vi "Updater Convert TDMS File 5.0 to 5.1 Prompted Input.vi"(6 "Connection Refnum In":T1, 7 "TDMS Path In":path, 8 "error in (no error)":errorcluster, 11 "TDMS File Ref":refnum<k34>) -> (0 "error out":errorcluster, 3 "TDMS File Ref":refnum<k34>, 4 "Connection Refnum Out":T1, 5 "TDMS Path Out":path)   [LabVIEW 2011]
uses:
  Summitek EXT/ODBC/SQL Controls/Connection Refnum.ctl
  server/database/Fields/Field Record.ctl
  server/database/Fields/Field DataTypes.ctl
  server/database/Fields/Field NextItem.ctl
  server/database/Fields/Field Order By.ctl
  Summitek EXT/OpenG EXT/file/file.llb/Convert File Extension (Path)__ogtk.vi
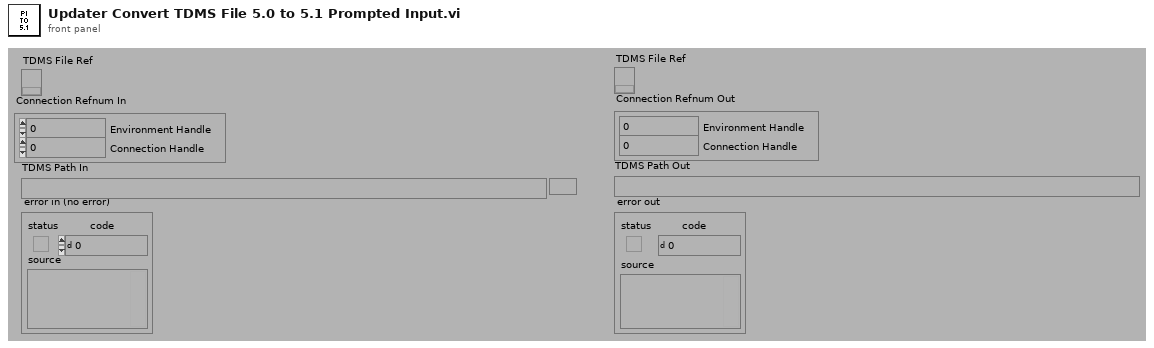
[diagram p1: front panel]
types:
  T1 = typedef "Connection Refnum.ctl" = cluster{"Environment Handle":i32, "Connection Handle":i32}
  T2 = enum16{"open", "open or create", "create or replace", "create", "open (read-only)"}
  T3 = typedef "Field Record.ctl" = cluster{"ixField":i32, "iSequenceOrder":i32, "sxFieldId":string, "sxSequenceId":string, "sDisplayName":string, "sValue":string, "sUnits":string, "nDataType":T4, "nNextItem":T5, "fSystem":bool, "fSystemValue":bool, "fRequired":bool, "fSetAtTest":bool, "fTestField":bool, "fDeleted":bool, "fIndexed":bool, "fFreeList":bool}
  T4 = typedef "Field DataTypes.ctl" = enum32{"text", "numeric", "list", "timestamp", "boolean"}
  T5 = typedef "Field NextItem.ctl" = enum32{"Reset", "Retain", "Auto-Increment"}
  T6 = typedef "Field Order By.ctl" = enum32{"sxSequenceId", "sxFieldId", "sDisplayName", "sValue", "fSetAtTest", "fRequired", "nNextItem"}
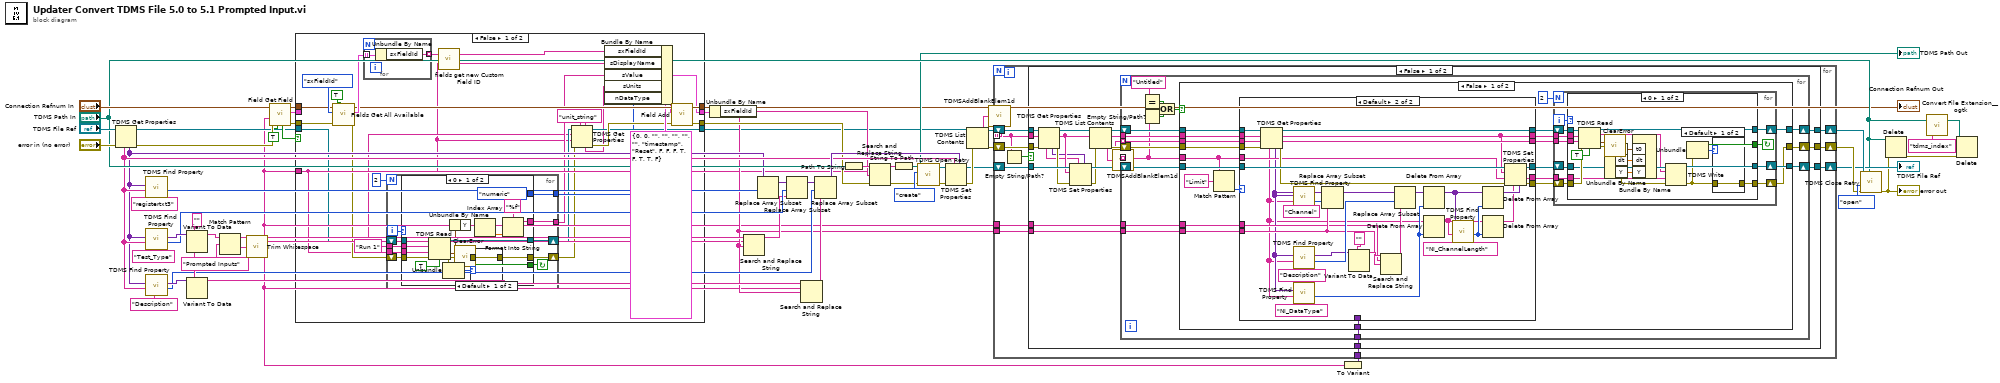
[diagram p0: block diagram]
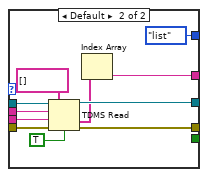
[diagram p3: hidden frame]
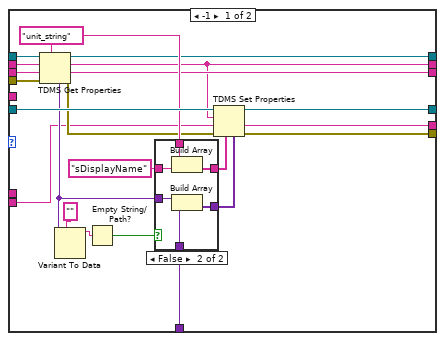
[diagram p5: hidden frame]
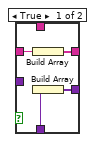
[diagram p6: hidden frame]
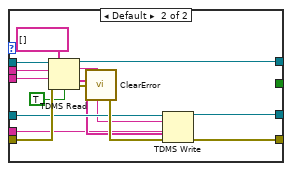
[diagram p8: hidden frame]
diagram:
  w2 = TRUE ("by sDisplayName? (f, by sFieldId)")
  w29 = "" ("element")
  n1 = TDMS Get Properties(8:"error in (no error)", 11:"TDMS File Ref") -> (0:w38:errorcluster, 3:w5:refnum<k34>, 4:w21:variant[], 6:w22:string[])  [unwired: 1 in, 5 out]
  n2 = call "TDMS Find Property.vi"("Property Name"="registertxt3" ("element"), "Property Names"=w22, "Property Values"=w21) -> ("Index"=w19:i32)  [unwired: 5 out]
  n3 = call "TDMS Find Property.vi"("Property Name"="Test_Type" ("element"), "Property Names"=w22, "Property Values"=w21) -> ("Index"=w18:i32, "Property Value"=w40:variant)  [unwired: 4 out]
  n4 = call "TDMS Find Property.vi"("Property Name"="Description" ("element"), "Property Names"=w22, "Property Values"=w21) -> ("Index"=w25:i32, "Property Value"=w30:variant)  [unwired: 4 out]
  n5 = Variant To Data(type=w29, Variant=w40) -> (data=w14:string)  [unwired: 1 in, 1 out]
  n6 = Variant To Data(type=w29, Variant=w30) -> (data=w28:string)  [unwired: 1 in, 1 out]
  n7 = Match Pattern(string=w14, regular expression="Prompted Inputs" ("element")) -> (after substring=w39:string)  [unwired: 4 out]
  n8 = call <vilib>:"Trim Whitespace.vi"("string"=w39) -> ("trimmed string"=w3:string)  [unwired: 1 in]
  n9 = call "Field Get Field.vi"("by sDisplayName? (f, by sFieldId)"=w2, "Include deleted? (F)"=w2, "error in (no error)"=w38, "sFieldId or sDisplayName (\"\")"=w3, "Connection Refnum"="Connection Refnum In") -> ("error out"=w11:errorcluster, "Field"=w36:T3, "Connection Refnum"=w10:T1, "Data Present?"=w12:bool)  [unwired: 1 in, 2 out]
  n10 = case shown="False" w12 {
    tunnel: w36 -> [_ w126]
    tunnel: [w60 w126] -> w6
    tunnel: w11 -> [w81 w127]
    tunnel: w10 -> [w82 w128]
    tunnel: [w75 w128] -> w8
    tunnel: [w74 w127] -> w9
    tunnel: w3 -> [w61 _]
    tunnel: w5 -> [w66 w125]
    tunnel: [w72 w125] -> w4
    frame False {
      w71 = "unit_string" ("string")
      w62 = "Run 1" ("group name in")
      w84 = TRUE
      n11 = call "Fields Get All Available.vi"("Combine All? (f)"=w84, "Include Deleted? (F)"=w84, "error in (no error)"=w81, "Sort by (sxSequenceId)"=Field_Order_By."sxFieldId" ("Sort by (Sequence_ID)"), "Connection Refnum"=w82) -> ("error out"=w63:errorcluster, "System or ALL Combined Fields"=w80:T3[], "Connection Refnum"=w78:T1)  [unwired: 1 in, 3 out]
      n12 = for {
        tunnel: w80 -> [w124] mode=indexing
        tunnel: [w123] -> w79 mode=indexing
        n13 = Unbundle By Name(w124) -> ("sxFieldId"=w123:string)
      }
      n14 = for {
        N: 2 -> [_]
        tunnel: w61 -> [w93]
        tunnel: w62 -> [w92]
        shift-right: [w94] -> w65
        shift-left: w66 -> [w91]
        tunnel: [w88] -> w68
        shift-right: [w86] -> w64
        shift-left: w63 -> [w87]
        tunnel: [w85] -> w67
        i -> [w90]
        stop <- w89 continue-if-true
        n15 = case shown="0" w90 {
          tunnel: [w111 w122] -> w94
          tunnel: w93 -> [w110 w121]
          tunnel: w92 -> [w109 w120]
          tunnel: w91 -> [w108 w119]
          tunnel: [w106 _] -> w89
          tunnel: [Field_DataTypes."numeric" ("nDataType") Field_DataTypes."list" ("nDataType")] -> w88
          tunnel: w87 -> [w104 w115]
          tunnel: [w103 w115] -> w86
          tunnel: [w98 w114] -> w85
          frame 0 {
            n16 = TDMS Read(0:w108, 5:w109, 7:w110, 11:w104, 13:TRUE ("return channels in file order? (F)")) -> (4:w111:refnum<k34>, 10:w97:waveform(dbl), 15:w96:errorcluster)  [unwired: 3 in, 3 out]
            n17 = Unbundle By Name(w97) -> ("Y"=w101:dbl[])
            n18 = call <vilib>:"ClearError.vi"("error in (no error)"=w96) -> ("error out"=w105:errorcluster)
            n19 = Unbundle(w105) -> ("status"=w106:bool, "code"=w107:i32)  [unwired: 1 out]
            n20 = case shown="Default" w107 {
              tunnel: [w112 _] -> w103
              tunnel: w105 -> [w112 _]
              frame Default {
              }
              frame -2525 {
              }
            }
            n21 = Index Array(array=w101) -> (element=w100:dbl)  [unwired: 1 in]
            n22 = Format Into String(format string="%f", w100) -> (resulting string=w98:string)  [unwired: 2 in, 1 out]
          }
          frame Default {
            n23 = TDMS Read(0:w119, 5:w120, 7:w121, 12:string[] [], 13:TRUE ("return channels in file order? (F)")) -> (4:w122:refnum<k34>, 10:w116:string[])  [unwired: 3 in, 4 out]
            n24 = Index Array(array=w116) -> (element=w114:string)  [unwired: 1 in]
          }
        }
      }
      n25 = call "fields get new Custom Field ID.vi"("Existing Field IDs (empty)"=w79) -> ("Custom Field ID"=w76:string)  [unwired: 1 in, 1 out]
      n26 = TDMS Get Properties(5:w71, 7:w71, 8:w64, 9:w61, 10:w62, 11:w65) -> (0:w73:errorcluster, 3:w72:refnum<k34>, 4:w70:string)  [unwired: 3 out]
      n27 = Bundle By Name(cluster=T3 {"ixField"=0, "iSequenceOrder"=0, "sxFieldId"="", "sxSequenceId"="", "sDisplayName"="", "sValue"="", "sUnits"="", "nDataType"=enum."timestamp", "nNextItem"=enum."Reset", "fSystem"=FALSE, "fSystemValue"=FALSE, "fRequired"=FALSE, "fSetAtTest"=TRUE, "fTestField"=FALSE, "fDeleted"=TRUE, "fIndexed"=TRUE, "fFreeList"=FALSE} ("Field Record"), "sxFieldId"=w76, "sDisplayName"=w61, "sValue"=w67, "sUnits"=w70, "nDataType"=w68) -> (w60:T3)
      n28 = call "Field Add.vi"("error in (no error)"=w73, "Field Record"=w60, "Connection Refnum"=w78) -> ("error out"=w74:errorcluster, "Connection Refnum"=w75:T1)  [unwired: 1 in, 6 out]
    }
    frame True {
    }
  }
  "Connection Refnum Out" <- w8
  n29 = Unbundle By Name(w6) -> ("sxFieldId"=w7:string)
  n30 = Search and Replace String(input string=w14, search string=w3, replace string=w7) -> (result string=w13:string)  [unwired: 1 in, 7 out]
  n31 = Replace Array Subset(array=w21, new element=w13, index=w19) -> (w20:variant[])
  n32 = Replace Array Subset(array=w20, new element=w13, index=w18) -> (w27:variant[])
  n33 = Search and Replace String(input string=w28, search string=w3, replace string=w7) -> (result string=w26:string)  [unwired: 1 in, 7 out]
  n34 = Replace Array Subset(array=w27, new element=w26, index=w25) -> (w24:variant[])
  n35 = Path To String(path="TDMS Path In") -> (string=w35:string)
  n36 = Search and Replace String(input string=w35, search string=w3, replace string=w7, error in=w9) -> (result string=w34:string, error out=w33:errorcluster)  [unwired: 6 out]
  n37 = String To Path(string=w34) -> (path=w15:path)
  "TDMS Path Out" <- w15
  n38 = call "TDMS Open Retry.vi"("error in (no error)"=w33, "Operation (0:open)"=T2."create" ("operation (0:open)"), "Path"=w15) -> ("error out"=w53:errorcluster, "TDMS File Ref"=w52:refnum<k34>)  [unwired: 1 in, 6 out]
  n39 = TDMS Set Properties(5:w24, 7:w22, 8:w53, 11:w52) -> (0:w57:errorcluster, 3:w51:refnum<k34>)  [unwired: 4 out]
  n40 = TDMS List Contents(4:w57, 7:w4) -> (0:w56:errorcluster, 2:w1:string[], 3:w50:refnum<k34>)  [unwired: 2 out]
  n41 = call <vilib>:"TDMSAddBlankElem1d.vi"("input string array"=w1) -> ("output string array with blank element at the beginning"=w59:string[])
  n42 = To Variant(anything=w3) -> (Variant=w16:variant)
  n43 = for {
    shift-right: [w137] -> w55
    shift-left: w56 -> [w138]
    tunnel: w59 -> [w136] mode=indexing
    shift-right: [w133] -> w49
    shift-left: w50 -> [w139]
    shift-right: [w132] -> w45
    shift-left: w51 -> [w135]
    tunnel: w16 -> [w131]
    tunnel: w7 -> [w130]
    tunnel: w3 -> [w129]
    n44 = Empty String/Path?(string/path=w136) -> (empty?=w134:bool)
    n45 = case shown="False" w134 {
      tunnel: w139 -> [w161 w318]
      tunnel: w138 -> [w160 w319]
      tunnel: [w153 w319] -> w137
      tunnel: w136 -> [w159 _]
      tunnel: w135 -> [w150 w317]
      tunnel: [w156 w318] -> w133
      tunnel: [w155 w317] -> w132
      tunnel: w131 -> [w143 _]
      tunnel: w130 -> [w142 _]
      tunnel: w129 -> [w141 _]
      frame False {
        n46 = TDMS Get Properties(8:w160, 10:w159, 11:w161) -> (0:w147:errorcluster, 2:w148:string, 3:w158:refnum<k34>, 4:w146:variant[], 6:w145:string[])  [unwired: 1 in, 3 out]
        n47 = TDMS Set Properties(5:w146, 7:w145, 8:w147, 10:w148, 11:w150) -> (0:w149:errorcluster, 3:w151:refnum<k34>)  [unwired: 3 out]
        n48 = TDMS List Contents(4:w149, 6:w148, 7:w158) -> (0:w154:errorcluster, 1:w140:string[], 2:w152:string, 3:w157:refnum<k34>)
        n49 = call <vilib>:"TDMSAddBlankElem1d.vi"("input string array"=w140) -> ("output string array with blank element at the beginning"=w144:string[])
        n50 = for {
          shift-right: [w170] -> w156
          shift-left: w157 -> [w175]
          shift-right: [w172] -> w155
          shift-left: w151 -> [w177]
          shift-right: [w171] -> w153
          shift-left: w154 -> [w176]
          tunnel: w152 -> [w174]
          tunnel: w144 -> [w173] mode=indexing
          tunnel: w144 -> [w164] mode=indexing
          tunnel: w143 -> [w165]
          tunnel: w142 -> [w163]
          tunnel: w141 -> [w162]
          n51 = Equal?(x="Untitled" ("string"), y=w164) -> (x = y?=w167:bool)
          n52 = Empty String/Path?(string/path=w164) -> (empty?=w168:bool)
          n53 = Or(x=w167, y=w168) -> (x .or. y?=w166:bool)
          n54 = case shown="False" w166 {
            tunnel: w177 -> [w198 w315]
            tunnel: w176 -> [w197 w314]
            tunnel: w175 -> [w196 w316]
            tunnel: w174 -> [w195 _]
            tunnel: w173 -> [w194 _]
            tunnel: [w191 w315] -> w172
            tunnel: [w190 w314] -> w171
            tunnel: [w189 w316] -> w170
            tunnel: w164 -> [w183 _]
            tunnel: w165 -> [w188 _]
            tunnel: w163 -> [w180 _]
            tunnel: w162 -> [w179 _]
            frame False {
              n55 = Match Pattern(string=w183, regular expression="Limit") -> (offset past match=w181:i32)  [unwired: 4 out]
              n56 = case shown="Default" w181 {
                tunnel: w198 -> [w220 w265]
                tunnel: w197 -> [w219 w264]
                tunnel: w196 -> [w218 w263]
                tunnel: w195 -> [w217 w262]
                tunnel: w194 -> [w216 w261]
                tunnel: [w215 w260] -> w193
                tunnel: [w214 w259] -> w192
                tunnel: w188 -> [w210 _]
                tunnel: [w203 w257] -> w187
                tunnel: [w202 w256] -> w186
                tunnel: [w201 w255] -> w185
                tunnel: w183 -> [_ w254]
                tunnel: w180 -> [w200 w245]
                tunnel: w179 -> [_ w244]
                tunnel: [w199 w231] -> w178
                frame -1 {
                  w208 = "unit_string" ("string")
                  n57 = TDMS Get Properties(7:w208, 8:w219, 9:w216, 10:w217, 11:w218) -> (0:w204:errorcluster, 1:w203:string, 2:w202:string, 3:w201:refnum<k34>, 4:w207:variant)  [unwired: 2 out]
                  n58 = Variant To Data(type="" ("element"), Variant=w207) -> (data=w212:string)  [unwired: 1 in, 1 out]
                  n59 = Empty String/Path?(string/path=w212) -> (empty?=w211:bool)
                  n60 = case shown="False" w211 {
                    tunnel: [w224 w228] -> w206
                    tunnel: w210 -> [w223 w230]
                    tunnel: [w222 w227] -> w205
                    tunnel: "sDisplayName" ("element") -> [w221 w229]
                    tunnel: w208 -> [_ w226]
                    tunnel: w207 -> [_ w225]
                    frame True {
                      n61 = Build Array(w221) -> (w224:string[])
                      n62 = Build Array(w223) -> (w222:variant[])
                    }
                    frame False {
                      n63 = Build Array(w226, w229) -> (w228:string[])
                      n64 = Build Array(w225, w230) -> (w227:variant[])
                    }
                  }
                  n65 = TDMS Set Properties(5:w205, 7:w206, 8:w204, 9:w200, 10:w202, 11:w220) -> (0:w215:errorcluster, 1:w199:string, 3:w214:refnum<k34>)  [unwired: 1 out]
                }
                frame Default {
                  n66 = TDMS Get Properties(8:w264, 9:w261, 10:w262, 11:w263) -> (0:w258:errorcluster, 1:w257:string, 2:w256:string, 3:w255:refnum<k34>, 4:w239:variant[], 6:w236:string[])  [unwired: 2 out]
                  n67 = call "TDMS Find Property.vi"("Property Name"="Channel" ("element"), "Property Names"=w236, "Property Values"=w239) -> ("Index"=w252:i32)  [unwired: 5 out]
                  n68 = call "TDMS Find Property.vi"("Property Name"="Description" ("element"), "Property Names"=w236, "Property Values"=w239) -> ("Index"=w249:i32, "Property Value"=w247:variant)  [unwired: 4 out]
                  n69 = call "TDMS Find Property.vi"("Property Name"="NI_DataType" ("element"), "Property Names"=w236, "Property Values"=w239) -> ("Index"=w238:i32)  [unwired: 5 out]
                  n70 = Replace Array Subset(array=w239, new element=w245, index=w252) -> (w250:variant[])
                  n71 = Variant To Data(type="" ("element"), Variant=w247) -> (data=w246:string)  [unwired: 1 in, 1 out]
                  n72 = Search and Replace String(input string=w246, search string=w244, replace string=w245) -> (result string=w243:string)  [unwired: 1 in, 7 out]
                  n73 = Replace Array Subset(array=w250, new element=w243, index=w249) -> (w242:variant[])
                  n74 = Delete From Array(array=w242, index=w238) -> (array with subset deleted=w233:variant[])  [unwired: 1 in, 1 out]
                  n75 = Delete From Array(array=w236, index=w238) -> (array with subset deleted=w232:string[])  [unwired: 1 in, 1 out]
                  n76 = call "TDMS Find Property.vi"("Property Name"="NI_ChannelLength" ("element"), "Property Names"=w232, "Property Values"=w233) -> ("Index"=w234:i32)  [unwired: 5 out]
                  n77 = Delete From Array(array=w233, index=w234) -> (array with subset deleted=w237:variant[])  [unwired: 1 in, 1 out]
                  n78 = Delete From Array(array=w232, index=w234) -> (array with subset deleted=w235:string[])  [unwired: 1 in, 1 out]
                  n79 = TDMS Set Properties(5:w237, 7:w235, 8:w258, 9:w254, 10:w256, 11:w265) -> (0:w260:errorcluster, 1:w231:string, 3:w259:refnum<k34>)  [unwired: 1 out]
                }
              }
              n80 = for {
                N: 2 -> [_]
                tunnel: w187 -> [w272]
                tunnel: w186 -> [w271]
                shift-right: [w268] -> w190
                shift-left: w193 -> [w276]
                shift-right: [w274] -> w191
                shift-left: w192 -> [w275]
                shift-right: [w273] -> w189
                shift-left: w185 -> [w270]
                tunnel: w178 -> [w266]
                i -> [w269]
                stop <- w267 continue-if-true
                n81 = case shown="0" w269 {
                  tunnel: w276 -> [w297 w313]
                  tunnel: w275 -> [w295 w311]
                  tunnel: [w293 w308] -> w274
                  tunnel: [w288 w307] -> w268
                  tunnel: [w292 w306] -> w273
                  tunnel: w272 -> [w291 w305]
                  tunnel: w271 -> [w290 w304]
                  tunnel: w270 -> [w289 w303]
                  tunnel: [w285 _] -> w267
                  tunnel: w266 -> [w284 w301]
                  frame 0 {
                    n82 = TDMS Read(0:w289, 5:w290, 7:w291, 11:w297, 13:TRUE ("return channels in file order? (F)")) -> (4:w292:refnum<k34>, 6:w294:string, 10:w283:waveform(dbl), 15:w278:errorcluster)  [unwired: 3 in, 2 out]
                    n83 = call <vilib>:"ClearError.vi"("error in (no error)"=w278) -> ("error out"=w296:errorcluster)
                    n84 = Unbundle By Name(w283) -> ("t0"=w282:timestamp, "dt"=w281:dbl, "Y"=w280:dbl[])
                    n85 = Bundle By Name("t0"=w282, "dt"=w281, "Y"=w280) -> (w279:waveform(dbl))  [unwired: 1 out]
                    n86 = TDMS Write(0:w295, 5:w294, 7:w284, 9:w279, 11:w296) -> (4:w293:refnum<k34>, 15:w286:errorcluster)  [unwired: 1 in, 2 out]
                    n87 = Unbundle(w286) -> ("status"=w285:bool, "code"=w287:i32)  [unwired: 1 out]
                    n88 = case shown="Default" w287 {
                      tunnel: [w298 _] -> w288
                      tunnel: w286 -> [w298 _]
                      frame Default {
                      }
                      frame -2525 {
                      }
                    }
                  }
                  frame Default {
                    n89 = TDMS Read(0:w303, 5:w304, 7:w305, 11:w313, 12:string[] [], 13:TRUE ("return channels in file order? (F)")) -> (4:w306:refnum<k34>, 6:w309:string, 10:w310:string[], 15:w300:errorcluster)  [unwired: 2 in, 2 out]
                    n90 = call <vilib>:"ClearError.vi"("error in (no error)"=w300) -> ("error out"=w312:errorcluster)
                    n91 = TDMS Write(0:w311, 5:w309, 7:w301, 9:w310, 11:w312) -> (4:w308:refnum<k34>, 15:w307:errorcluster)  [unwired: 1 in, 2 out]
                  }
                }
              }
            }
            frame True {
            }
          }
        }
      }
      frame True {
      }
    }
  }
  "TDMS File Ref" <- w45
  n92 = call "TDMS Close Retry.vi"("TDMS Path"="TDMS Path In", "error in (no error)"=w55, "Operation (0:open)"=T2."open" ("operation (0:open)"), "TDMS File Ref"=w49) -> ("error out"=w44:errorcluster)  [unwired: 1 in, 6 out]
  "error out" <- w44
  n93 = Delete(path (use dialog)="TDMS Path In", error in=w44) -> (error out=w48:errorcluster)  [unwired: 5 out]
  n94 = call-poly "Convert File Extension__ogtk.vi"("new ending (none)"="tdms_index", "file name"="TDMS Path In") -> ("new filename"=w47:path)  [unwired: 1 out]
  n95 = Delete(path (use dialog)=w47, error in=w48) -> ()  [unwired: 6 out]
